vi "transreg.vi"() -> ()   [LabVIEW 2021]
panel:
  out "output trans string":string
  out "input string 2":string
  out "input string":string
  in  "enter your string, bro":string
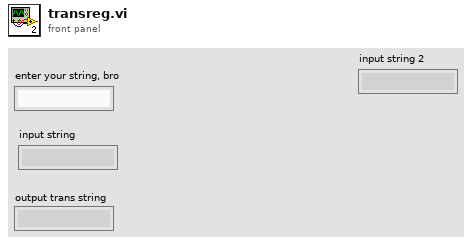
[diagram p1: front panel]
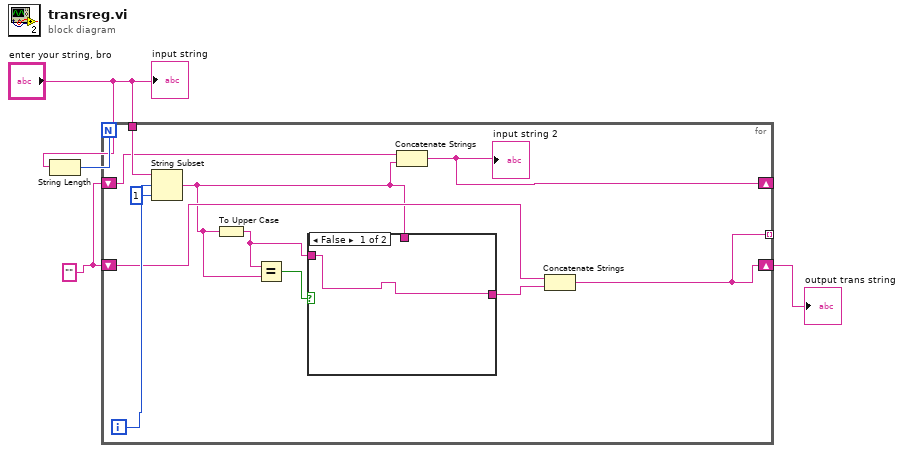
[diagram p0: block diagram]
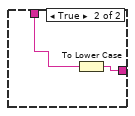
[diagram p2: hidden frame]
diagram:
  w1 = "" ("string")
  n1 = String Length(string="enter your string, bro") -> (length=w4:i32)
  n2 = for {
    N: w4 -> [_]
    tunnel: "enter your string, bro" -> [w12]
    shift-right: [w9] -> w2
    shift-left: w1 -> [w10]
    tunnel: [w9] -> _ mode=indexing
    shift-right: [w6] -> _
    shift-left: w1 -> [w8]
    i -> [w11]
    n3 = String Subset(string=w12, offset (0)=w11, length (rest)=1 ("length (rest)")) -> (substring=w7:string)
    n4 = To Upper Case(1:w7) -> (0:w15:string)
    n5 = Equal?(x=w15, y=w7) -> (x = y?=w14:bool)
    n6 = case shown="False" w14 {
      tunnel: w7 -> [_ w17]
      tunnel: [w16 w18] -> w13
      tunnel: w15 -> [w16 _]
      frame False {
      }
      frame True {
        n7 = To Lower Case(string=w17) -> (all lower case string=w18:string)
      }
    }
    n8 = Concatenate Strings(w8, w7) -> (w6:string)
    "input string 2" <- w6
    n9 = Concatenate Strings(w10, w13) -> (w9:string)
  }
  "output trans string" <- w2
  "input string" <- "enter your string, bro"
